vi "TouchSensor.vi"() -> ()   [LabVIEW 2016, in "ENED1100-UCBA-Sensor-Motor-Testing.lvrbt"]
uses:
  ENED1100-UCBA-Sensor-Motor-Testing.lvrbt
  <vilib>/NXT/Subs/LVHSConnector.ctl
  <vilib>/NXT/LegoClasses/BrickReference/BrickReference.lvclass
  <vilib>/NXT/Block Support/NXT_InputPort.ctl
  <vilib>/NXT/Dual Mode Library/Sensors/Touch_Pressed.vi
  <vilib>/NXT/Dual Mode Library/Sound/PlayD.vi
panel:
  out "NXT/EV3 2":T1
  in  "Tone (440 Hz)":u16=440
  in  "Select the Active Port for the sensor":T2 items=["Port 1", "Port 2", "Port 3", "Port 4"]
  in  "NXT/EV3":T1
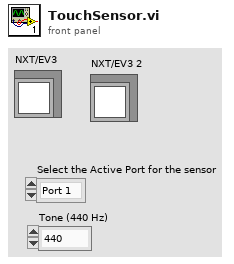
[diagram p1: front panel]
types:
  T1 = typedef "LVHSConnector.ctl" = refnum<class "BrickReference.lvclass">
  T2 = typedef "NXT_InputPort.ctl" = u32
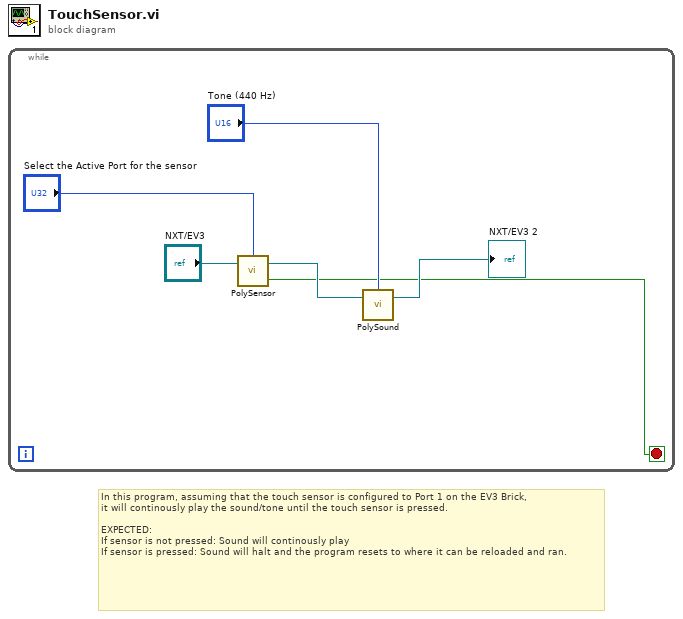
[diagram p0: block diagram]
diagram:
  # "In this program, assuming that the touch sensor is configured to Port 1 on the EV3 Brick,\nit will continously play the sound/tone until the touch sensor is pressed.\n\nEXPECTED:\nIf sensor is not pressed: Sound will continously play\nIf sensor is pressed: Sound will halt and the program resets to where it can be reloaded and ran."
  n1 = while {
    stop <- w1 stop-if-true
    n2 = call-poly <vilib>:"PolySensor.vi"("NXT/EV3"="NXT/EV3", "Port (Port 1)"="Select the Active Port for the sensor") -> ("Yes / No"=w1:bool, "NXT/EV3"=w4:T1)  [unwired: 1 in]
    n3 = call-poly <vilib>:"PolySound.vi"("NXT/EV3"=w4, "Octave"="Tone (440 Hz)") -> ("NXT/EV3"=→"NXT/EV3 2":T1)  [unwired: 2 in]
  }
